vi "SP Command.vi"(8 "error in (no error)":errorcluster, 10 "power limit value":u32, 11 "PSP-405 resource in":refnum<visa-resource-name>) -> (0 "error out":errorcluster, 3 "PSP-405 resource out":refnum<visa-resource-name>)   [LabVIEW 2017, in "GW Instek PSP-405.lvlib"]
doc: "The SP command sets the power limit. When the power limit is changed the current limit will be automatically altered to suit."
uses:
  GW Instek PSP-405.lvlib
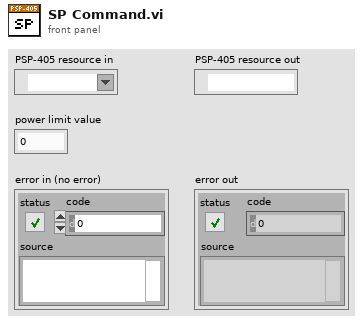
[diagram p1: front panel]
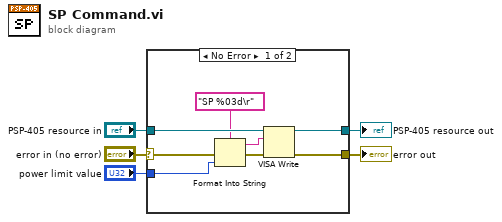
[diagram p0: block diagram]
diagram:
  n1 = case shown="No Error" "error in (no error)" {
    selector: "error in (no error)" -> [w9 w15]
    tunnel: "PSP-405 resource in" -> [w12 w14]
    tunnel: [w13 w15] -> w4
    tunnel: [w11 w14] -> w2
    tunnel: "power limit value" -> [w7 _]
    frame No Error {
      n2 = Format Into String(format string="SP %03d\r", error in=w9, w7) -> (resulting string=w10:string, error out=w8:errorcluster)  [unwired: 1 in]
      n3 = VISA Write(VISA resource name=w12, write buffer=w10, error in (no error)=w8) -> (VISA resource name out=w11:refnum<visa-resource-name>, error out=w13:errorcluster)  [unwired: 1 out]
    }
    frame Error {
    }
  }
  "error out" <- w4
  "PSP-405 resource out" <- w2
